vi "RSNRPZ Get Trigger Slope.vi"(8 "error in (no error)":errorcluster, 10 "Channel (1)":i32=1, 11 "VISA session":refnum<visa-resource-name> caption="VISA resource name") -> (0 "error out":errorcluster, 2 "Trigger Slope":i32, 3 "dup VISA session":refnum<visa-resource-name> caption="VISA resource name")   [LabVIEW 2010]
doc: "This VI reads whether the rising (POSitive) or the falling (NEGative) edge of the signal is used for triggering.\n\nRemote-control command(s):\nTRIG:SLOP?"
uses:
  rsnrpz_32.dll
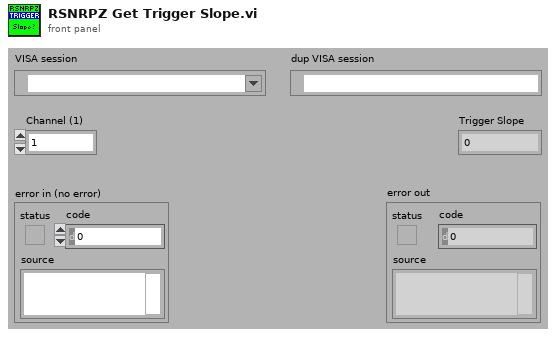
[diagram p1: front panel]
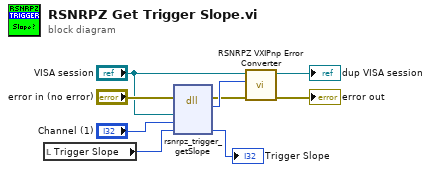
[diagram p0: block diagram]
diagram:
  n1 = local read "Trigger Slope"() -> (w7:i32)
  n2 = dll-call lib="rsnrpz_32.dll" fn="rsnrpz_trigger_getSlope"(error in="error in (no error)", "VISA Session"="VISA session", "Channel"="Channel (1)", "Trigger Slope"=w7) -> (error out=w5:errorcluster, "Status"=w9:i32, "Trigger Slope"=→"Trigger Slope":i32)  [unwired: 4 in, 1 out]
  n3 = call <instrlib>:"RSNRPZ VXIPnp Error Converter.vi"("error in"=w5, "VXIPnp error code"=w9, "VISA session"="VISA session") -> ("error out"=→"error out":errorcluster, "dup VISA session"=→"dup VISA session":refnum<visa-resource-name>)  [unwired: 7 in]
